vi "CloseInstrument.vi"(8 "error in (no error)":errorcluster, 11 "reference in":refnum<class "niMmWave_Reciever.lvclass">) -> (0 "error out":errorcluster, 3 "reference out":refnum<class "niMmWave_Reciever.lvclass">)   [LabVIEW 2019, in "niMmWave_Reciever.lvclass"]
doc: "Closes all instrument resources"
uses:
  niMmWave_Reciever.lvclass
  C:/Barkhausen mmWave radar/Development/LV/Barkhausen mmWave hardware control/Host/SubVIs/mmWave instrument_class/mmWave instrument.lvclass
  mmWave instrument_class/Instrument state.ctl
  mmWave HW Control/mmWave HW Control.lvlib
  mmWave instrument_class/mmWave instrument.lvclass
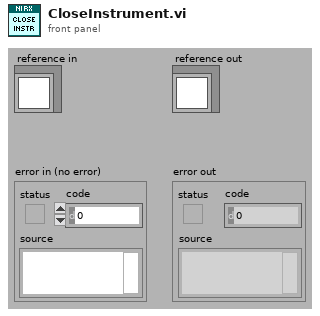
[diagram p1: front panel]
types:
  T1 = typedef "mmWave instrument.lvclass/Instrument state.ctl" = enum16{"Off", "Initialization", "Configuration", "Running", "Calibration"}
  T2 = typedef "niMmWave_Reciever.lvclass/ObjectAttributesRef.ctl" = refnum<data-value>
  T3 = typedef "niMmWave_Reciever.lvclass/ObjectAttributes.ctl" = cluster{"session":T4[], "HW.RX devices":T18, "RF config":T19, "RX trigger options":T20, "RX samples":i32, "RX Fs":dbl}
  T4 = typedef "Session.ctl" = cluster{"3620 session":refnum<queue>, "tx baseband session":T5, "rx baseband session":T13, "tx gain (dB)":dbl, "rx gain (dB)":dbl, "hardware configuration":T14, "gain ranging":T16[], "pxi trigger bus information":T17}
  T5 = typedef "Tx Baseband Session.ctl" = cluster{"3610 session":T6, "7902 reference":T12}
  T6 = typedef "ni3610_and_ni3630_Driver_Lib.lvlib/Main Settings.ctl" = cluster{"VISA resource name":refnum<visa-resource-name>, "Address Space":T7, "window_offset":u32, "register_addresses":T8, "required_MM_fpga_version":cluster{"signature":u32, "hardware":u32, "current revision":u32, "oldest revision":u32}, "CPLD Oldest Compat Version ":cluster{"hardware":u32, "CPLD firmware":u32}, "MM_FPGA_image_location":string, "is_init":bool, "card_type":T9, "DacLmkConfigFileName":string, "AdcLmkConfigFileName":string, "AdcConfigFileName":string, "DacConfigFileName_RevA":string, "DacConfigFileName_RevB":string, "Mulde hardware revision":u8, "bypass DAC PLL\n":bool, "IQ Card Revision":T10, "board capability":T11}
  T7 = typedef "VISA Register Access Address Space.ctl" = u16
  T8 = typedef "ni3610_and_ni3630_Driver_Lib.lvlib/Register Adresses.ctl" = cluster{"MM based Registers":cluster{"Revision":u32, "OldestCompatRev":u32, "signature":u32, "scratch":u32, "LedControl":u32, "BoardHwRev":u32, "BoardControl":u32, "ThermalStatus":u32, "BasebandStatus":u32, "BasebandControl":u32, "BasebandAuxSetup":u32, "BasebandAuxStatus":u32, "LmkSyncOutSetup":u32, " AdcSyncOutSetup":u32, " InjSyncOutSetup":u32, " PxiTrig0OutSetup":u32, " PxiTrig1OutSetup":u32, " PxiTrig2OutSetup":u32, " PxiTrig3OutSetup":u32, " PxiTrig4OutSetup":u32, " PxiTrig5OutSetup":u32, " PxiTrig6OutSetup":u32, " PxiTrig7OutSetup":u32}, "CPLD based Registers":cluster{"SlaveSignature":u32, "SlaveRevision":u32, "SlaveOldestCompatRev":u32, "SlaveScratch":u32, "SlaveSetup":u32, "SlaveStatus":u32, "IDacReg_offset":u32, "LMKRegGrp0_offset":u32, "QDacReg_offset":u32, "BrdTempSensorVal":u32, "TempSensorPowerDown":u32, "GPIOReg_offset":u32, "IAdcReg_offset":u32, "QAdcReg_offset":u32, "LMKRegGrp1_offset":u32, "QadcTempSensorVal":u32, "IadcTempSensorVal":u32, "RevisionReg":u32, "VcxoReg":u32, "CpldStatusReg":u32, "PowerReg":u32, "VBiasEnReg":u32, "ExtRefOeReg":u32, "QdacCtrlReg":u32, "QdacStatusReg":u32, "IdacCtrlReg":u32, "IdacStatusReg":u32, "QdacJtagIn":u32, "QdacJtagOut":u32, "IdacJtagIn":u32, "IdacJtagOut":u32, "IqDcSetupReg":u32, "QadcStatusReg":u32, "IadcStatusReg":u32, "BrdSetupReg":u32, "IqDcRevisionReg":u32, "PllStatusReg":u32, "EndpointScratchReg":u32, "AdcSyncCfgReg":u32, "IqCardOpampReg":u32}, "CPLD Register Offset":u32, "MM  Register Offset":u32, " PxiTrig0OutSetup":u32}
  T9 = typedef "ni3610_and_ni3630_Driver_Lib.lvlib/Base Card Type.ctl" = enum16{"unspecified", "ADC", "DAC"}
  T10 = typedef "ni3610_and_ni3630_Driver_Lib.lvlib/IQ Card Revision.ctl" = enum16{"RevA", "RevB", "RevC", "RevD"}
  T11 = typedef "ni3610_and_ni3630_Driver_Lib.lvlib/Board Capability.ctl" = cluster{"baseband sync":enum16{"no baseband sync", "baseband sync"}}
  T12 = typedef "Blank FPGA Reference.ctl" = refnum<k20>
  T13 = typedef "Rx Baseband Session.ctl" = cluster{"3630 session":T6, "7902 reference":T12}
  T14 = typedef "Hardware Configuration.ctl" = cluster{"direction":T15, "baseband only":bool}
  T15 = typedef "Direction.ctl" = enum16{"Transceiver", "Receiver", "Transmitter"}
  T16 = typedef "Gain Ranging.ctl" = cluster{"gain ranging active scope":string, "gain ranging stream session":refnum<k20>}
  T17 = typedef "PXI Trigger Bus Info.ctl" = cluster{"chassis resource name":refnum<visa-resource-name>, "7902R (TX)":i16, "3610 (TX)":i16, "3620 (IF)":i16, "3630 (RX)":i16, "7902R (RX)":i16}
  T18 = typedef "mmWave HW Control.lvlib/HW RX resources cluster.ctl" = cluster{"HW.IF":tag, "HW.ADC":refnum<visa-resource-name>, "HW.RX FPGA":tag}
  T19 = typedef "mmWave HW Control.lvlib/HW RX RF config cluster.ctl" = cluster{"Gain":dbl, "Frequency":dbl, "mmWave adapter":string}
  T20 = typedef "TX trigger config.ctl" = cluster{"delay":dbl, "trig source":T21, "PXI src":i32, "export":T22, "PXI dest":i32}
  T21 = typedef "FPGA Utility.lvlib/FPGA driver trigger source.ctl" = enum16{"Use Tclk", "PXI_Trig", "Aurora RX trig"}
  T22 = typedef "FPGA Utility.lvlib/FPGA driver trigger destination.ctl" = enum16{"None", "Source trig", "Synced trig", "Delayed sync"}
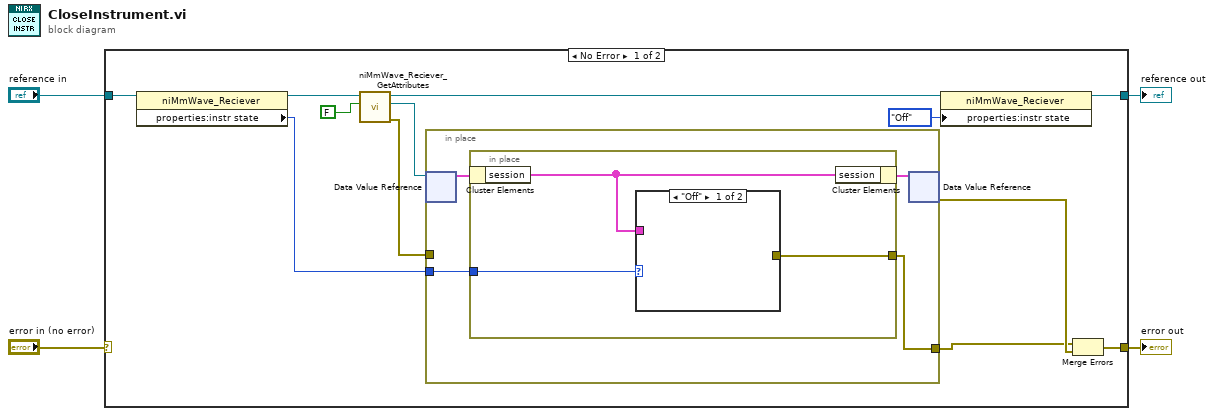
[diagram p0: block diagram]
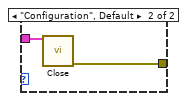
[diagram p2: hidden frame]
diagram:
  n1 = case shown="No Error" "error in (no error)" {
    selector: "error in (no error)" -> [_ w27]
    tunnel: [w16 w27] -> w3
    tunnel: [w6 w26] -> w1
    tunnel: "reference in" -> [w13 w26]
    frame No Error {
      n2 = property class="niMmWave_Reciever"(reference=w13) -> (reference out=w8:refnum<class "niMmWave_Reciever.lvclass">, "properties:instr state"=w7:T1)  [unwired: 1 in, 1 out]
      n3 = call "niMmWave_Reciever_GetAttributes.vi"("return data? (T)"=FALSE, "reference in"=w8) -> ("error out"=w11:errorcluster, "attributes ref"=w9:T2, "reference out"=w10:refnum<class "niMmWave_Reciever.lvclass">)  [unwired: 6 in, 1 out]
      n4 = in-place {
        in-place-border: w11 -> [_]
        in-place-border: [w18] -> w14
        in-place-border: w7 -> [w17]
        n5 = in-place-dvr #1(w9) -> (w19:T3)  [unwired: 1 out]
        n6 = in-place {
          in-place-border: [w22] -> w18
          in-place-border: w17 -> [w21]
          n7 = in-place-cluster #2(w19) -> ("session"=w23:T4[])
          n8 = case shown="\"Off\"" w21 {
            tunnel: w23 -> [_ w25]
            tunnel: [_ w24] -> w22
            frame "Off" {
            }
            frame "Configuration", Default {
              n9 = call "Close.vi"("session"=w25) -> ("error out"=w24:errorcluster)  [unwired: 14 in]
            }
          }
          n10 = in-place-cluster #2("session"=w23) -> (w20:T3)
        }
        n11 = in-place-dvr #1(w20) -> (w15:errorcluster)  [unwired: 1 out]
      }
      n12 = property class="niMmWave_Reciever"(reference=w10, "properties:instr state"=Instrument_state."Off" ("instr state")) -> (reference out=w6:refnum<class "niMmWave_Reciever.lvclass">)  [unwired: 1 in, 1 out]
      n13 = Merge Errors(w14, w15) -> (w16:errorcluster)
    }
    frame Error {
    }
  }
  "error out" <- w3
  "reference out" <- w1
